vi "Get GUI Item Value - Variant.vi"(7 "Default":variant, 8 "error in (no error)":errorcluster, 10 "FP Item Name":string, 11 "uService Template in":refnum<class "Father of all uServices.lvclass">) -> (0 "error out":errorcluster, 2 "Value":variant, 3 "uService Template out":refnum<class "Father of all uServices.lvclass">)   [LabVIEW 2026, in "TALOS.lvlib" / "Father of all uServices.lvlib" / "Father of all uServices.lvclass"]
uses:
  Father of all uServices.lvclass
  C:/LabVIEW Code/TALOS/talos/Ancestor/Ancestor/Ancestor.lvclass
  Ancestor/Ancestor/Ancestor.lvclass/Ancestor.ctl
  Classes/uService List/uService List.lvclass/uService List.ctl
  Classes/uService List/Get FP Items Refs Map.vi
  Ancestor/Ancestor/Read ID.vi
  Support VIs/Generate Error.vi
  FGV/Error Memory/Get Error Description.vi
  Support VIs/Get PC name.vi
  Support VIs/Get Class Name.vi
  <vilib>/Utility/error.llb/Clear Errors.vi
  FGV/Error Memory/Error Memory Core.vi
  <vilib>/AdvancedString/Delimited String to 1D String Array.vi
  <vilib>/AdvancedString/Delimited String to 1D String Array (string).vi
  Support VIs/Circus Root Path.vi
  FGV/Error Memory/Error Crt Lvl checker.vi
  FGV/Error Memory/Error Memory Core.vi/40c8088d-b597-4017-91af-faa98e00292e.vi
  FGV/Error Memory/Error Memory Core.vi/d4a3ab98-063c-4e44-b43d-fbdcfe6c2be2.vi
  Support VIs/Global Memory.vi
  <vilib>/Utility/LVClass/Get LV Class Name.vi
  Support VIs/Is in Packed Library.vi
  Support VIs/TALOS Root path.vi
  Support VIs/Read CSV worksheet.vi
  Support VIs/Global Constants.vi
  <vilib>/Utility/error.llb/General Error Handler.vi
  Support VIs/Error Log.vi
  Ancestor/Ancestor/Ancestor.lvclass
  <vilib>/Comparison/Equal/Equal Functor/Equal Functor.lvclass
  Classes/uService List/uService List.lvclass
  TALOS.lvlib
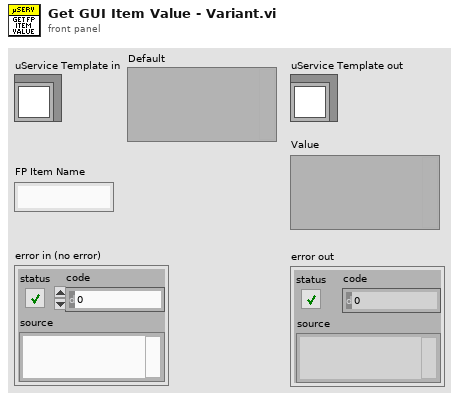
[diagram p1: front panel]
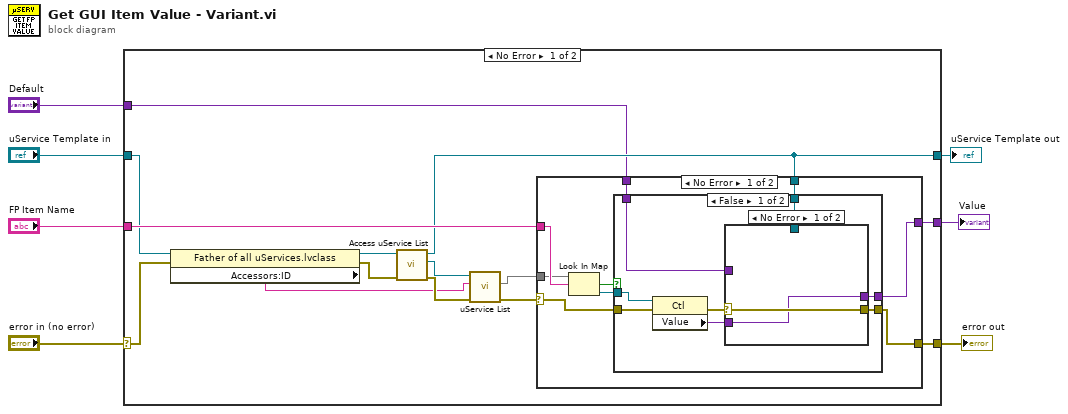
[diagram p0: block diagram]
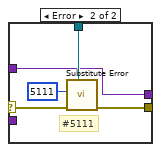
[diagram p2: hidden frame]
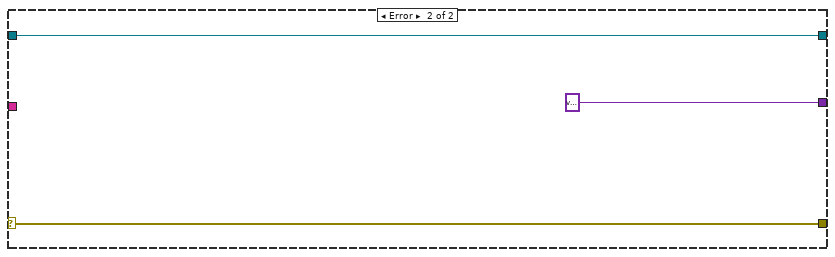
[diagram p5: hidden frame]
diagram:
  n1 = case shown="No Error" "error in (no error)" {
    selector: "error in (no error)" -> [w19 w52]
    tunnel: "uService Template in" -> [w13 w50]
    tunnel: [w21 variant ("Value")] -> w6
    tunnel: "FP Item Name" -> [w20 _]
    tunnel: [w18 w52] -> w3
    tunnel: [w9 w50] -> w2
    tunnel: "Default" -> [w8 _]
    frame No Error {
      n2 = property class="Father of all uServices.lvclass"(reference=w13, error in=w19) -> (reference out=w16:refnum<class "Father of all uServices.lvclass">, error out=w15:errorcluster, "Accessors:ID"=w11:string)
      n3 = call-dynamic "Access uService List.vi"("error in (no error)"=w15, "Ancestor in"=w16) -> ("error out"=w12:errorcluster, "uService List out"=w14:refnum<class "uService List.lvclass">, "Ancestor out"=w9:refnum<class "Father of all uServices.lvclass">)  [unwired: 7 in]
      n4 = call-poly "uService List.vi"("error in (no error)"=w12, "ID"=w11, "uService List in"=w14) -> ("error out"=w17:errorcluster, "FP Items Refs Map"=w10:map{string, refnum<vi>})  [unwired: 6 in, 1 out]
      n5 = case shown="No Error" w17 {
        selector: w17 -> [w25 w49]
        tunnel: [w28 w48] -> w21
        tunnel: w20 -> [w27 _]
        tunnel: [w26 w49] -> w18
        tunnel: w10 -> [w24 _]
        tunnel: w9 -> [w23 _]
        tunnel: w8 -> [w22 w48]
        frame No Error {
          n6 = Look In Map(map=w24, key=w27) -> (key not found?=w29:bool, value=w30:refnum<vi>)  [unwired: 1 in]
          n7 = case shown="False" w29 {
            tunnel: w30 -> [w37 _]
            tunnel: [w35 w47] -> w26
            tunnel: [w31 w46] -> w28
            tunnel: w25 -> [w38 w47]
            tunnel: w23 -> [w34 _]
            tunnel: w22 -> [w33 w46]
            frame False {
              n8 = property class="Ctl"(reference=w37, error in=w38) -> (error out=w36:errorcluster, "Value"=w32:variant)  [unwired: 1 out]
              n9 = case shown="No Error" w36 {
                selector: w36 -> [w40 w45]
                tunnel: [w40 w44] -> w35
                tunnel: w34 -> [_ w43]
                tunnel: w33 -> [_ w41]
                tunnel: w32 -> [w39 _]
                tunnel: [w39 w41] -> w31
                frame No Error {
                }
                frame Error {
                  # "#5111"
                  n10 = call "Substitute Error.vi"("LabVIEW Object"=w43, "error in (no error)"=w45, "Error Code"=5111) -> ("error out"=w44:errorcluster)  [unwired: 8 in]
                }
              }
            }
            frame True {
              # "Error/do nothing"
            }
          }
        }
        frame Error {
        }
      }
    }
    frame Error {
    }
  }
  "error out" <- w3
  "Value" <- w6
  "uService Template out" <- w2
